vi "set_Message.vi"(0 "HB_Dialog in":refnum<class "HB_Dialog.lvclass">, 7 "Message":string, 11 "error in (no error)":errorcluster) -> (4 "HB_Dialog out":refnum<class "HB_Dialog.lvclass">, 15 "error out":errorcluster)   [LabVIEW 2009, in "HB_Inherance_Example.lvlib" / "HB_Dialog.lvclass"]
doc: "Set message text."
uses:
  HB_Dialog.lvclass
  HB_Dialog.lvclass/HB_Dialog.ctl
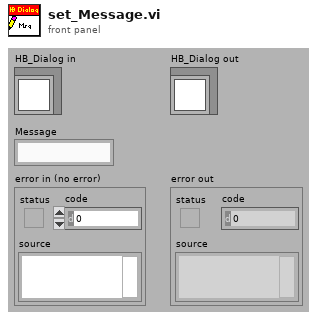
[diagram p1: front panel]
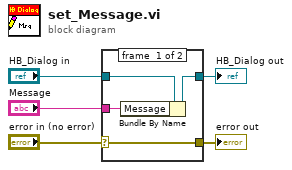
[diagram p0: block diagram]
diagram:
  n1 = case shown="No Error" "error in (no error)" {
    selector: "error in (no error)" -> [w9 w10]
    tunnel: [w9 w10] -> w4
    tunnel: [w7 w11] -> w2
    tunnel: "HB_Dialog in" -> [w8 w11]
    tunnel: "Message" -> [w6 _]
    frame #0 {
      n2 = Bundle By Name(cluster=w8, "Message"=w6) -> (w7:refnum<class "HB_Dialog.lvclass">)
    }
    frame #1 {
    }
  }
  "error out" <- w4
  "HB_Dialog out" <- w2
